vi "movimentacao_cin_inv_bezier_2_com_sensor_att.vi"() -> ()   [LabVIEW 2017]
doc: "The myRIO Project template acquires acceleration data from the onboard accelerometer and displays the changes of acceleration values in a waveform chart."
uses:
  <vilib>/Analysis/Matrix/Datatypes/RealMatrix.ctl
  <vilib>/myRIO/Instrument Drivers/Onboard IO/I2C/typedefs/I2C User Configuration.ctl
  <vilib>/myRIO/Instrument Drivers/Onboard IO/I2C/typedefs/I2C Transfer Rate.ctl
  <vilib>/myRIO/Instrument Drivers/Onboard IO/PWM/typedefs/PWM Reference.ctl
  <vilib>/myRIO/Common/Instrument Driver Framework/Utilities/typedefs/myRIO Generic Hardware Reference.ctl
  <vilib>/myRIO/Common/Instrument Driver Framework/Utilities/typedefs/Hardware Version Enum.ctl
  <vilib>/myRIO/Common/Instrument Driver Framework/Utilities/typedefs/myRIO v1.0 Reference.ctl
  <vilib>/myRIO/Common/Instrument Driver Framework/Utilities/typedefs/Generic FPGA Reference.ctl
  <vilib>/myRIO/Common/Instrument Driver Framework/myRIO v1.0/PWM/typedefs/PWM Channels Enum.ctl
  <vilib>/myRIO/Instrument Drivers/Onboard IO/PWM/typedefs/PWM Configuration.ctl
  <vilib>/userdefined/High Color/nirio_resource_hc.ctl
  <vilib>/myRIO/Instrument Drivers/Onboard IO/I2C/typedefs/I2C Reference.ctl
  <vilib>/myRIO/Common/Instrument Driver Framework/myRIO v1.0/I2C/typedefs/I2C Channels Enum.ctl
  <vilib>/myRIO/Instrument Drivers/Onboard IO/I2C/typedefs/I2C Configuration.ctl
  <vilib>/myRIO/Common/Instrument Driver Framework/myRIO v1.0/I2C/vis/myRIO v1.1 Open I2C.vi
  <vilib>/myRIO/Common/Instrument Driver Framework/myRIO v1.0/PWM/vis/myRIO v1.1 Open PWM.vi
  <vilib>/myRIO/Common/Instrument Driver Framework/Utilities/vis/Validate Channels.vi
  <vilib>/myRIO/Common/Instrument Driver Framework/myRIO v1.0/I2C/vis/myRIO v1.0 Reserve I2C.vi
  <vilib>/myRIO/Common/Instrument Driver Framework/myRIO v1.0/I2C/vis/myRIO v1.0 Close I2C.vi
  <vilib>/myRIO/Common/Instrument Driver Framework/myRIO v1.0/PWM/vis/myRIO v1.0 Reserve PWM.vi
  <vilib>/myRIO/Instrument Drivers/Onboard IO/PWM/vis/Set Duty Cycle and Frequency.vi
  <vilib>/myRIO/Common/Instrument Driver Framework/myRIO v1.0/PWM/vis/myRIO v1.0 Close PWM.vi
  <vilib>/myRIO/Common/Instrument Driver Framework/myRIO v1.0/I2C/vis/myRIO v1.0 Build MUX Configuration I2C.vi
  <vilib>/myRIO/Common/Instrument Driver Framework/myRIO v1.0/Resource Manager/vis/myRIO v1.0 Reserve Channel List.vi
  <vilib>/myRIO/Common/Instrument Driver Framework/myRIO v1.0/I2C/vis/myRIO v1.0 Unreserve I2C.vi
  <vilib>/myRIO/Common/Instrument Driver Framework/myRIO v1.0/PWM/vis/myRIO v1.0 Build MUX Configuration PWM.vi
  <vilib>/myRIO/Common/Instrument Driver Framework/myRIO v1.0/PWM/vis/myRIO v1.0 Unreserve PWM.vi
  <vilib>/myRIO/Common/Instrument Driver Framework/myRIO v1.0/Resource Manager/vis/myRIO v1.0 Create Configuration List.vi
  <vilib>/myRIO/Common/Instrument Driver Framework/myRIO v1.0/Resource Manager/vis/myRIO v1.0 Reserve Channel.vi
  <vilib>/myRIO/Common/Instrument Driver Framework/myRIO v1.0/Resource Manager/vis/myRIO v1.0 Unreserve Channel.vi
  <vilib>/myRIO/Common/Instrument Driver Framework/myRIO v1.0/Resource Manager/vis/myRIO v1.0 Unreserve Channel List.vi
  <vilib>/myRIO/Common/Instrument Driver Framework/myRIO v1.0/Resource Manager/vis/myRIO v1.0 Build Mutex Name.vi
  <vilib>/Utility/VariantDataType/GetNumericInfo.vi
  <vilib>/Utility/error.llb/Error Cluster From Error Code.vi
  <vilib>/myRIO/Common/Instrument Driver Framework/myRIO v1.0/myRIO v1.1 Open.vi
  <vilib>/myRIO/Common/Instrument Driver Framework/Utilities/vis/IO Manager.vi
  <vilib>/myRIO/Common/Instrument Driver Framework/Utilities/vis/Configuration Manager.vi
  <vilib>/myRIO/Common/Instrument Driver Framework/myRIO v1.0/Resource Manager/vis/myRIO v1.0 Configure IO.vi
  <vilib>/myRIO/Common/Instrument Driver Framework/myRIO v1.0/myRIO v1.0 Close.vi
  <vilib>/myRIO/Common/Instrument Driver Framework/myRIO v1.0/PWM/vis/myRIO v1.0 Write PWM.vi
  <vilib>/myRIO/Common/Instrument Driver Framework/myRIO v1.0/PWM/vis/myRIO v1.0 Shutdown PWM.vi
  <vilib>/myRIO/Common/Instrument Driver Framework/myRIO v1.0/I2C/vis/myRIO v1.0 Configure I2C.vi
  <vilib>/myRIO/Common/Instrument Driver Framework/myRIO v1.0/I2C/vis/myRIO v1.0 Shutdown I2C.vi
  <vilib>/myRIO/Instrument Drivers/Onboard IO/PWM/vis/myRIO PWM Open.xnode
  <vilib>/myRIO/Instrument Drivers/Onboard IO/I2C/vis/myRIO I2C Open.xnode
  <vilib>/myRIO/Instrument Drivers/Onboard IO/PWM/PWM.lvlib
  <vilib>/myRIO/Instrument Drivers/Onboard IO/I2C/I2C.lvlib
  <vilib>/Analysis/Matrix/NI_Matrix.lvlib
panel:
  out "x-y":i32
  out "Fim_manipulacao":bool
  out "indexador 2":i32
  in  "Time Target (s) 2":dbl=0.2 format="%#_13g"
  out "x < y?":bool
  out "reconheceu 2":bool
  out "Local_da_peca 2":i8
  out "Elapsed Time (s) 2":dbl
  out "Time has Elapsed 2":bool
  out "x .and. y?":bool
  out "var aux":bool=TRUE
  in  "OK Button":bool
  out "Detectou 2":bool
  out "mean out":dbl
  in  "y":dbl=135.0
  out "PARAR ESTEIRA":bool
  out "reconheceu":bool
  out "x .and. y? 2":bool
  out "Detectou":bool
  in  "Duty Cycle Abert 2":dbl=0.08 format="%#_13g"
  out "Local_da_peca":i8
  out "PARAR 2":bool
  out "spreadsheet string":string
  out "error out 2":errorcluster
  out "init status 2":bool
  out "did_timeout 2":bool
  out "dt 2":u32
  out "Waveform Chart 2":u16(graph)
  out "Range (cm)":u16
  out "objeto":bool
  out "distancaia 2":dbl format="%0.2f"
  out "result string":string
  out "iterador":u32
  out "number of rows":i32
  out "matrix":T1
  out "subarray":dbl[](array[numeric])
  out "appended array 2":dbl[](array[numeric])
  out "POS_E_ORIEN_HOME":dbl[](array[numeric])
  out "ANG_POSI_E_ORIEN_HOME":dbl[](array[numeric])
  out "CURRENT POSITIONS OF THE MOTORS":dbl[](array[numeric])
  in  "angulo_garra":dbl(knob) scale=-180.0..180.0
  in  "Duty Cycle Abert":dbl=0.04 format="%#_13g"
  out "Actuator 2":bool
  in  "Actuator":bool
  in  "Conveyor speed (mm/s)":dbl(slide)=200.0 step=1.0 scale=0.0..350.0
  out "indexador":i32
  out "Manipulando":bool
  out "Está em Home":bool
  out "Posicao_desejada":bool
  in  "Home":bool
  in  "error in (no error)":errorcluster
  in  "PARAR":bool
  in  "POSITION VECTOR":dbl[](array[numeric])
  # "ROTINA DE CONTROLE DO PROTÓTIPO DE FMS"
  # "COMANDO DE POSI敲O\nATUAL DOS MOTORES"
  # "OPERATION STATUS"
  # "ÂNGULOS DE JUNTAS"
  # "THETA 1"
  # "MOTOR 1"
  # "HOME"
  # "THETA 2"
  # "MOTOR 2"
  # "POSI敲O DESEJADA"
  # "THETA 3"
  # "MOTOR 3"
  # "OBJETO DETECTADO"
  # "THETA 4"
  # "MOTOR 4"
  # "MANIPULANDO"
  # "THETA 5"
  # "MOTOR 5"
  # "ESTEIRA PARADA"
  # "MOTOR 6"
  # "ATUADOR"
  # "VELOCIDADE DA ESTEIRA (mm/s)"
  # "0,042"
  # "SCL- CINZA - 32\nSDA - ROXO - 34\nTERRA - BRANCO\nVCC - PRETO"
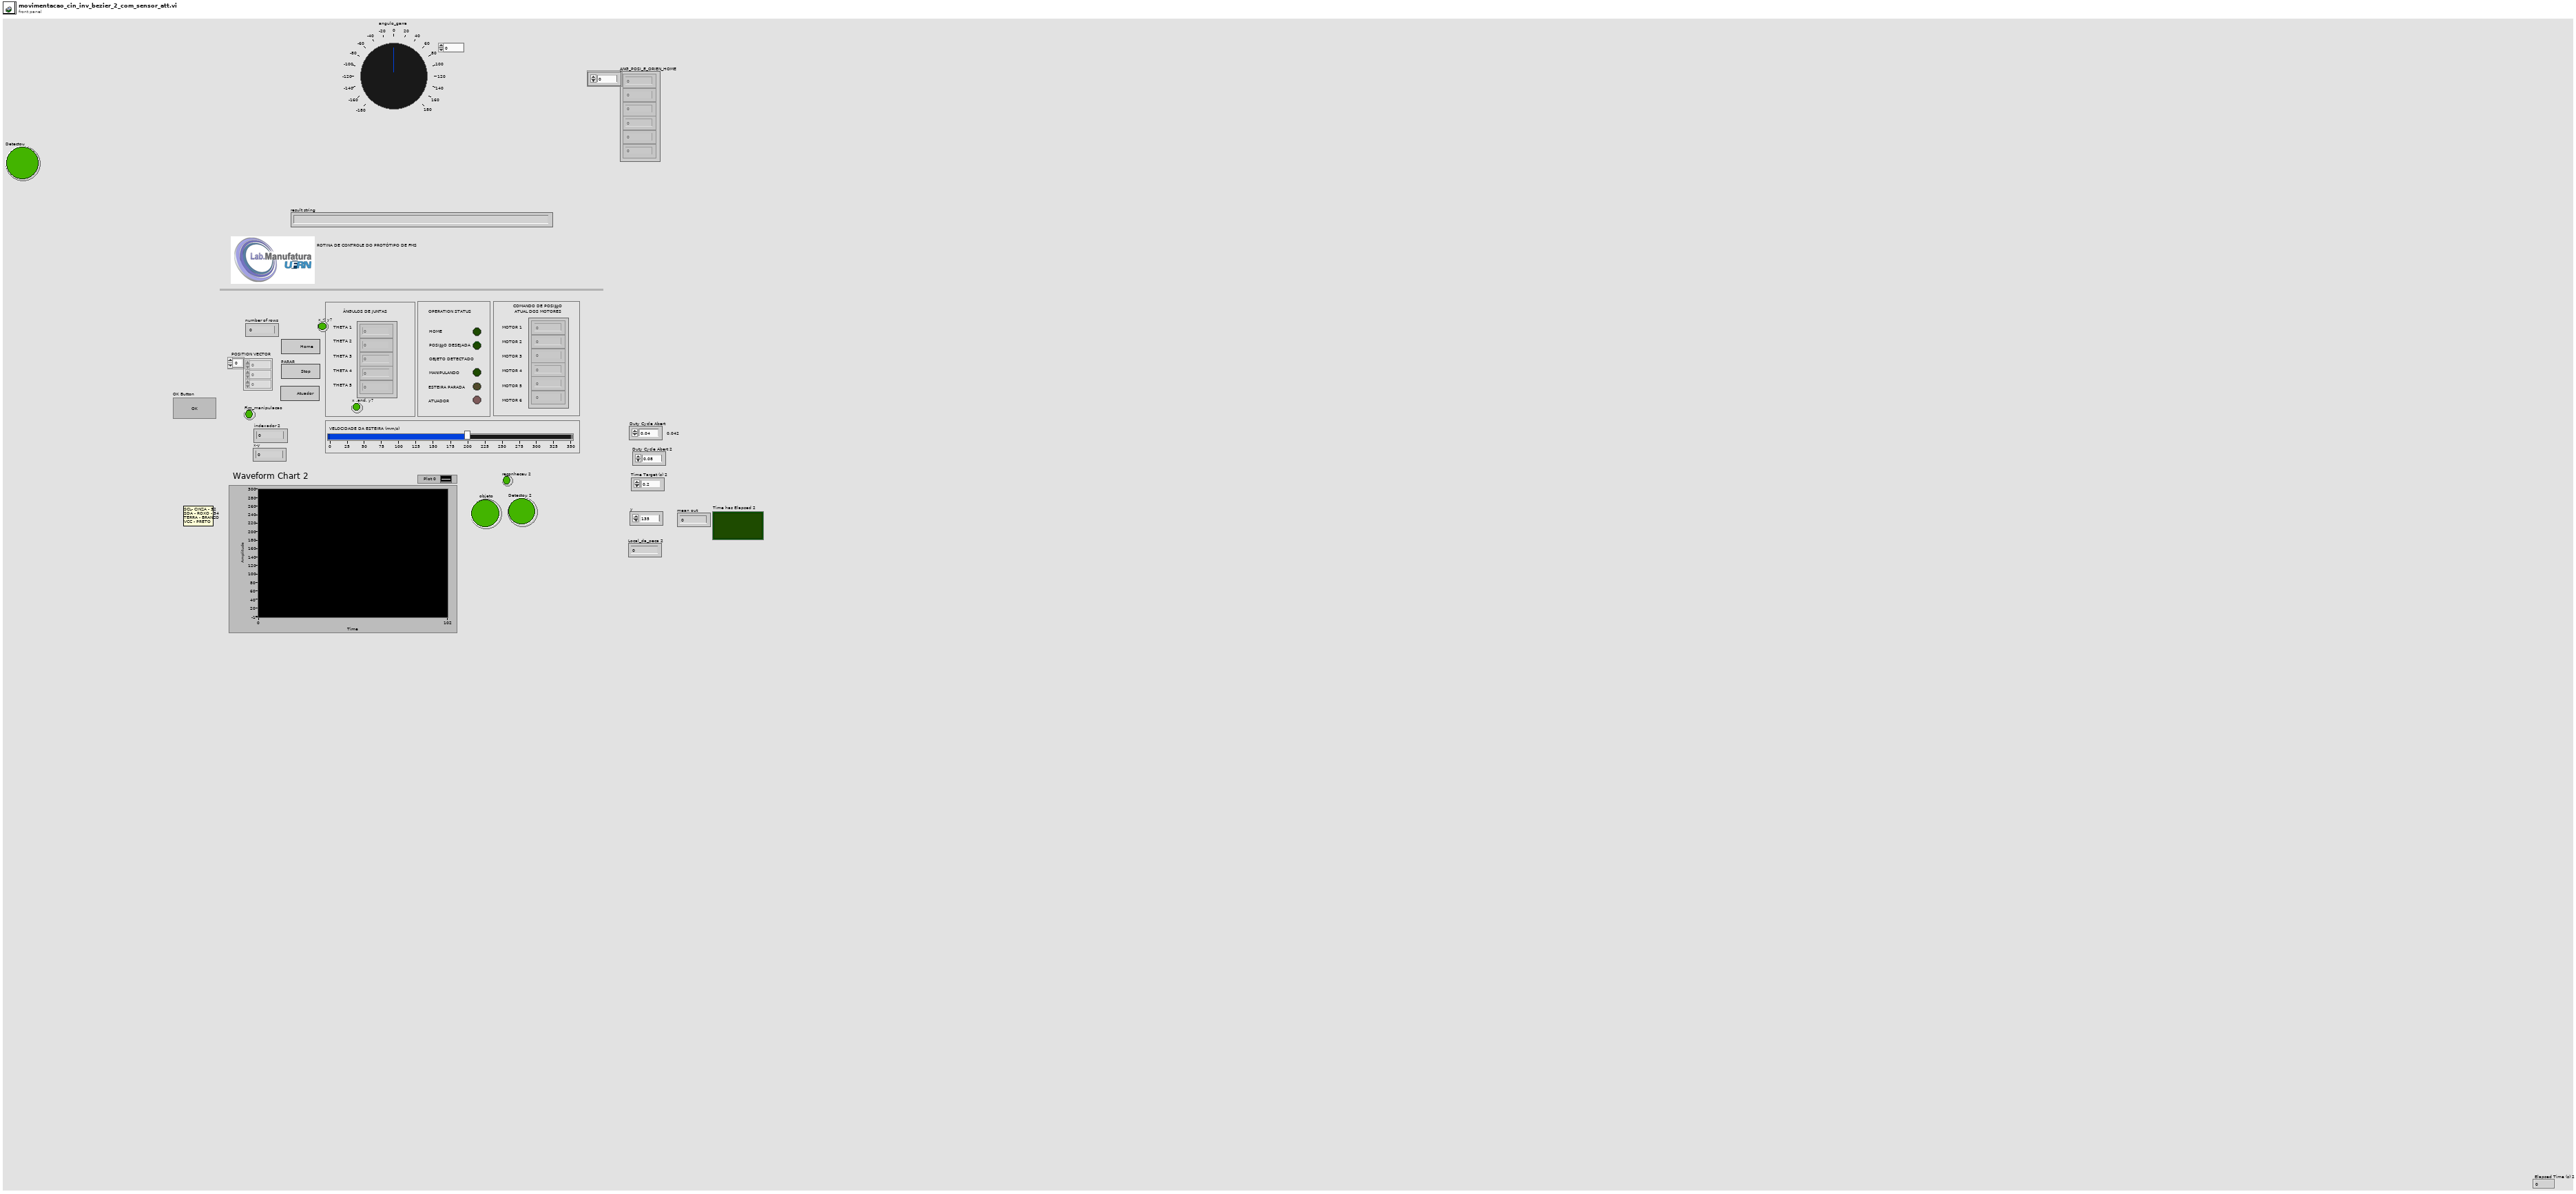
[diagram p1: front panel]
types:
  T1 = typedef "NI_Matrix.lvlib/RealMatrix.ctl" = dbl[][]
  T2 = typedef "I2C.lvlib/I2C User Configuration.ctl" = cluster{"I2C Transfer Rate":T3}
  T3 = typedef "I2C.lvlib/I2C Transfer Rate.ctl" = enum16{"Standard mode (100 kbps)", "Fast mode (400 kbps)"}
  T4 = cluster{"theta 1":dbl, "theta 2":dbl, "theta 3":dbl, "theta5":dbl, "theta4":dbl}
  T5 = typedef "nirio_resource_hc.ctl" = tag
  T6 = typedef "Hardware Version Enum.ctl" = enum16{"Unknown", "myRIO-1900", "myRIO-1950", "roboRIO", "NI ELVIS RIO CM"}
  T7 = typedef "PWM.lvlib/PWM Reference.ctl" = cluster{"myRIO Reference":T8, "PWM Channels Enum":T11, "PWM Configuration":T12}
  T8 = typedef "myRIO Generic Hardware Reference.ctl" = cluster{"myRIO Model":T6, "myRIO Hardware Reference":T9}
  T9 = typedef "myRIO v1.0 Reference.ctl" = cluster{"Generic FPGA Reference":T10, "Allow multiple opens":bool}
  T10 = typedef "Generic FPGA Reference.ctl" = refnum<k20>
  T11 = typedef "PWM Channels Enum.ctl" = enum16{"Not Connected", "C/PWM0", "C/PWM1", "A/PWM0", "A/PWM1", "A/PWM2", "B/PWM0", "B/PWM1", "B/PWM2", "PWM/PWM0", "PWM/PWM1", "PWM/PWM2", "PWM/PWM3", "PWM/PWM4", "PWM/PWM5", "PWM/PWM6", "PWM/PWM7", "PWM/PWM8", "PWM/PWM9"}
  T12 = typedef "PWM.lvlib/PWM Configuration.ctl" = cluster{"Frequency":dbl, "Duty Cycle":dbl}
  T13 = typedef "I2C.lvlib/I2C Reference.ctl" = cluster{"myRIO Reference":T8, "I2C Channels Enum":T14, "I2C Configuration":T15}
  T14 = typedef "I2C Channels Enum.ctl" = enum16{"Not Connected", "A/I2C", "B/I2C", "I2C/I2C"}
  T15 = typedef "I2C.lvlib/I2C Configuration.ctl" = cluster{"I2C Transfer Rate":T3}
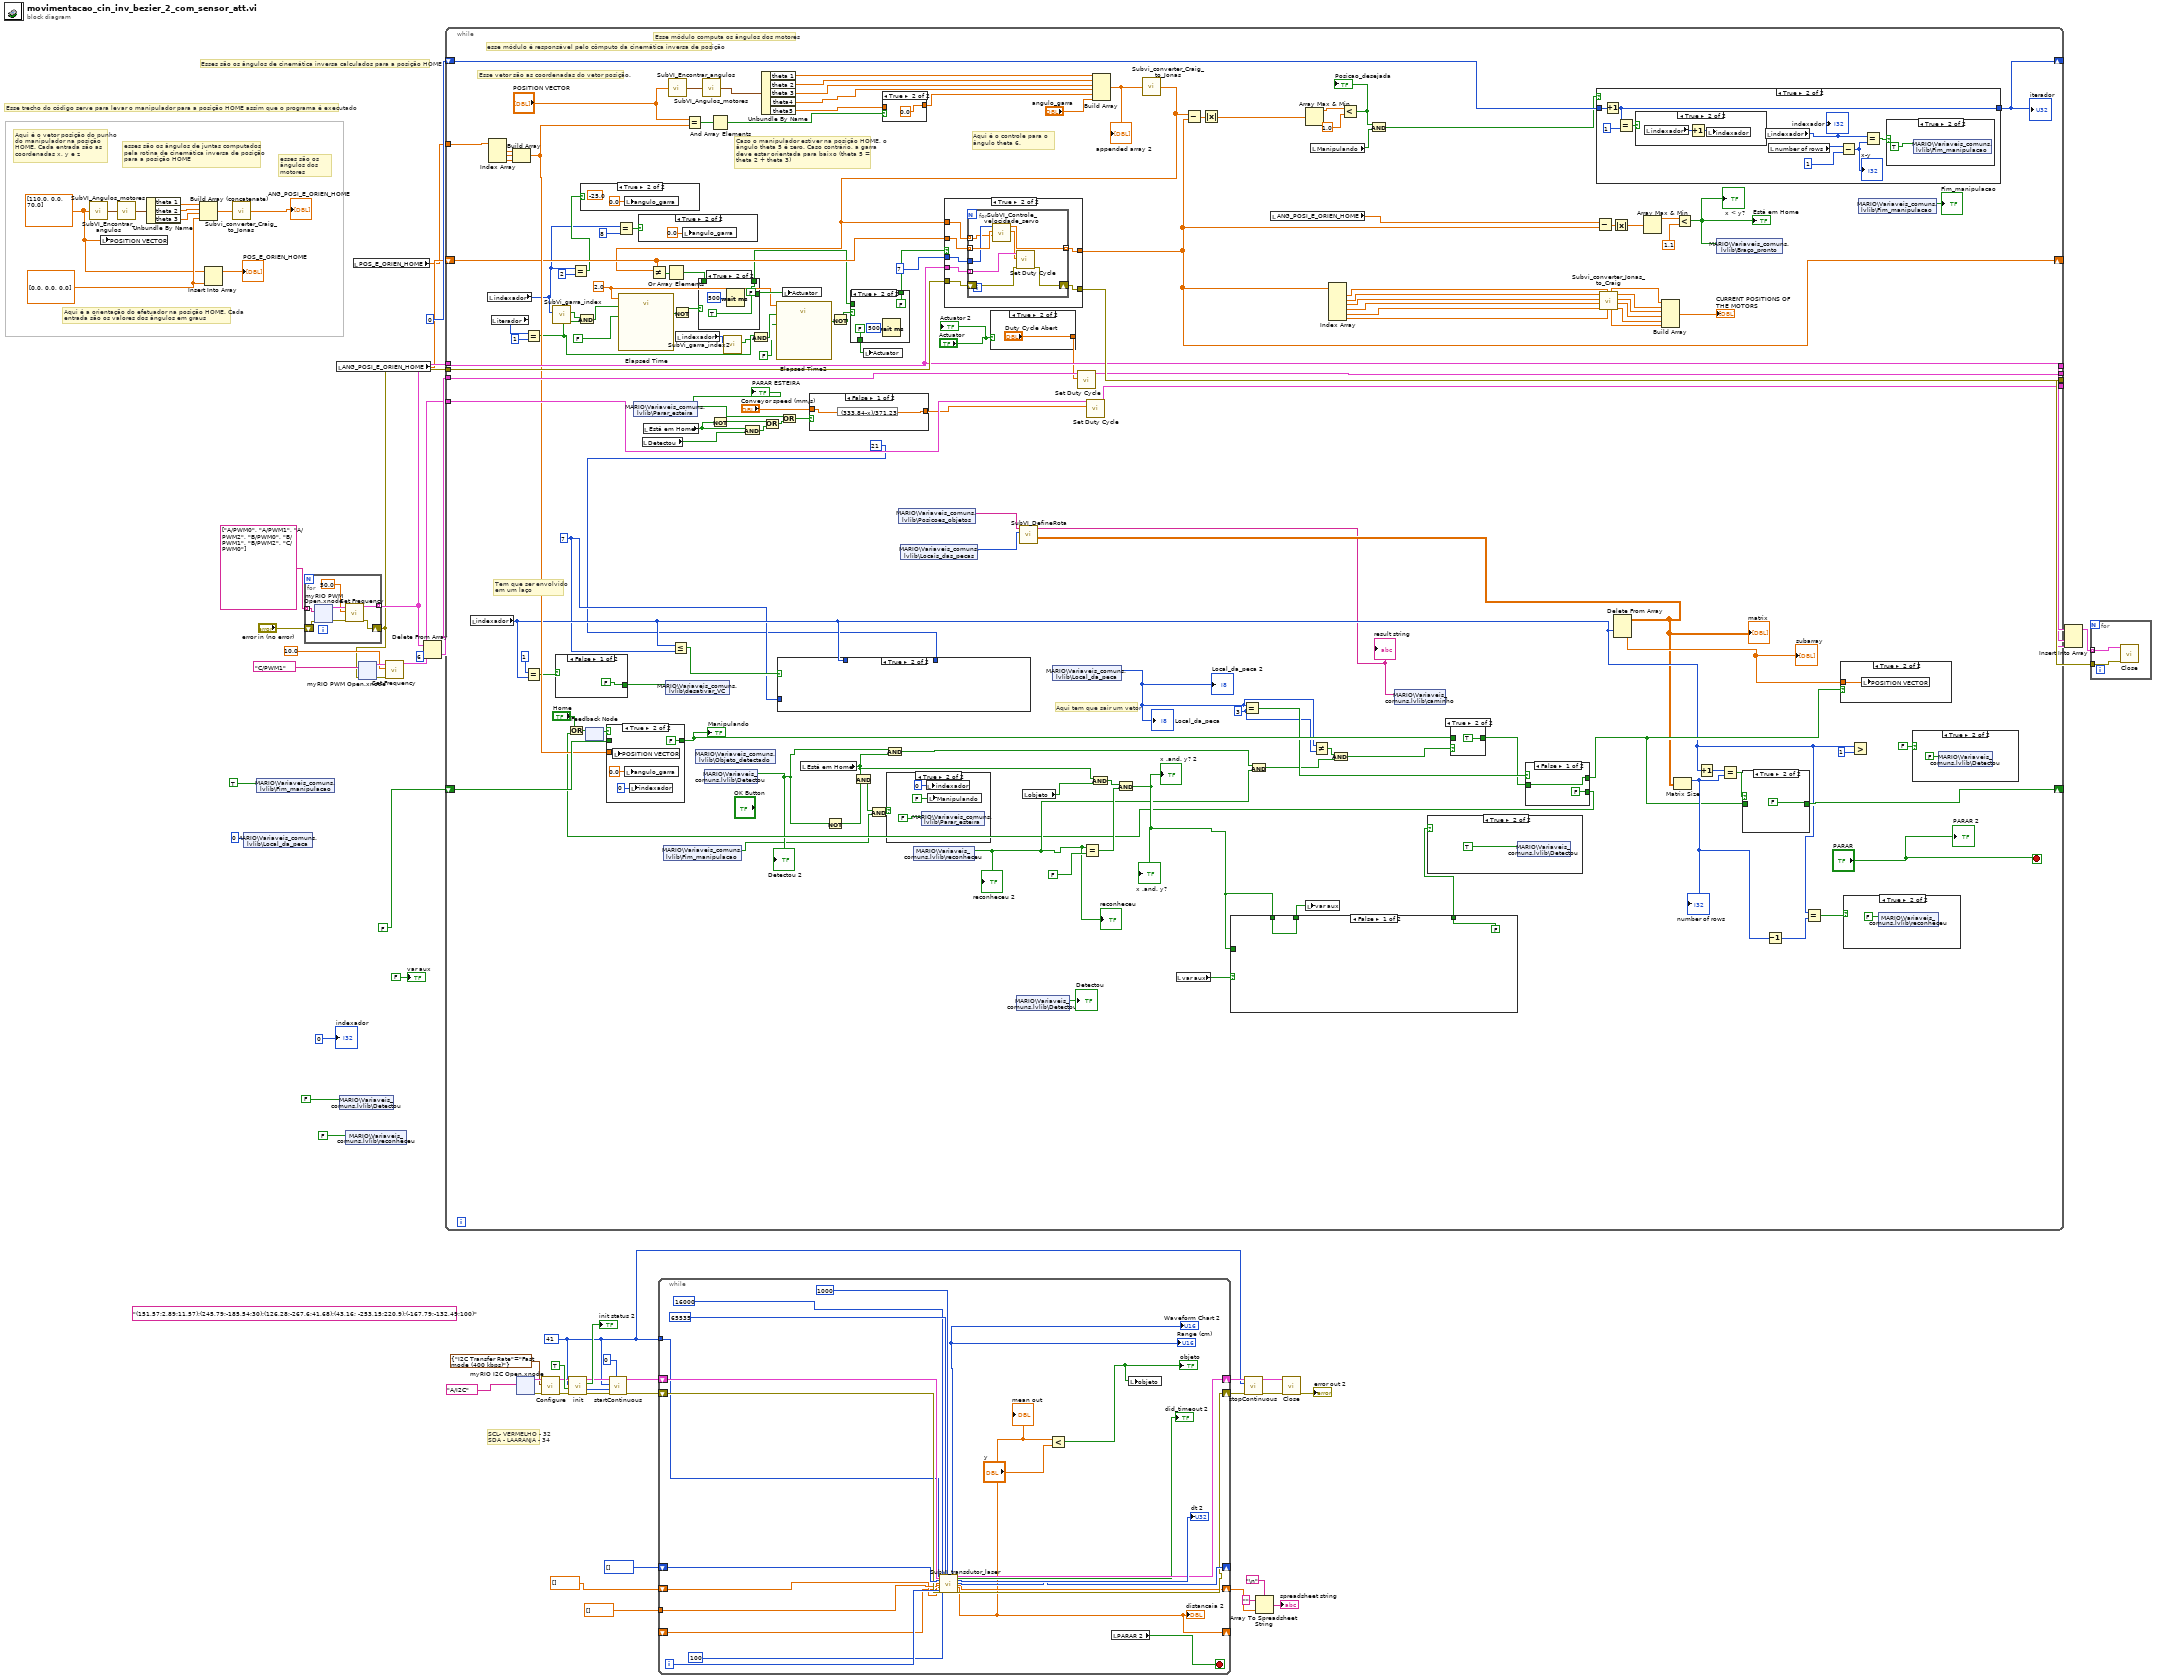
[diagram p0: block diagram]
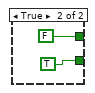
[diagram p2: hidden frame]
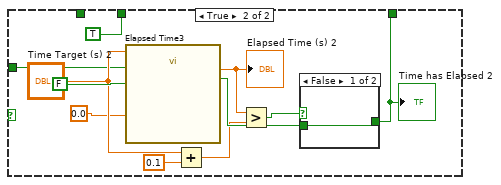
[diagram p3: hidden frame]
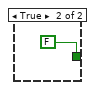
[diagram p4: hidden frame]
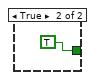
[diagram p8: hidden frame]
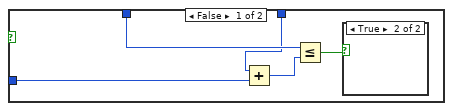
[diagram p11: hidden frame]
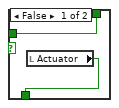
[diagram p13: hidden frame]
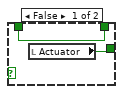
[diagram p14: hidden frame]
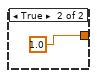
[diagram p16: hidden frame]
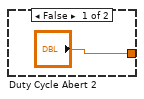
[diagram p17: hidden frame]
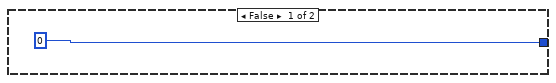
[diagram p20: hidden frame]
diagram:
  w13 = u8 41
  (unwired) "(151,57;2,89;11,57);(245,79;-185,54;30);(126,28;-267,6;41,68);(43,16; -253,15;220,9);(-167,79;-132,49;100)" ("String 2")
  w40 = dbl[] [0.0, 0.0, 0.0] ("vetor_P")
  w3 = dbl[] [110.0, 0.0, 70.0] ("vetor_P")
  # "esses são os ângulos dos motores"
  # "esses são os ângulos de juntas computados pela rotina de cinemática inversa de posição para a posição HOME"
  # "Esses são os ângulos de cinemática inversa calculados para a posição HOME"
  # "Aqui é a orientação do efetuador na posição HOME. Cada entrada são os valores dos ângulos em graus"
  # "Aqui é o vetor posição do punho do manipulador na posição HOME. Cada entrada são as coordenadas x, y e z"
  # "Esse trecho do código serve para levar o manipulador para a posição HOME assim que o programa é executado"
  # "SCL- VERMELHO - 32\nSDA - LAARANJA - 34"
  n1 = call "SubVI_Encontrar_angulos.vi"("vetor_P"=w3) -> ("ângulos de Juntas"=w35:T4)
  n2 = local write "POSITION VECTOR"(w3) -> ()
  n3 = call "SubVI_Angulos_motores.vi"("input cluster"=w35) -> ("output cluster"=w34:T4)
  n4 = Unbundle By Name(w34) -> ("theta 1"=w44:dbl, "theta 2"=w43:dbl, "theta 3"=w42:dbl)
  n5 = Build Array (concatenate)(w44, w43, w42, w40) -> (w37:dbl[])
  n6 = Insert Into Array(array=w3, new element=w40) -> (→"POS_E_ORIEN_HOME":dbl[])  [unwired: 1 in]
  n7 = call "Subvi_converter_Craig_to_Jonas.vi"("array"=w37) -> ("appended array"=→"ANG_POSI_E_ORIEN_HOME":dbl[])
  n8 = shared-variable "MARIO\\Variaveis_comuns.lvlib\\Local_da_peca"(i8 0 ("Local_da_peca")) -> ()  [unwired: 1 in, 1 out]
  n9 = shared-variable "MARIO\\Variaveis_comuns.lvlib\\Fim_manipulacao"(TRUE) -> ()  [unwired: 1 in, 1 out]
  n10 = for {
    tunnel: tag[] ["A/PWM0", "A/PWM1", "A/PWM2", "B/PWM0", "B/PWM1", "B/PWM2", "C/PWM0"] -> [w67] mode=indexing
    tunnel: [w66] -> w57 mode=indexing
    shift-right: [w65] -> w46
    shift-left: "error in (no error)" -> [w64]
    n11 = xnode ("myRIO PWM Open.xnode")("error in (no error)"=w64, "Channel Name"=w67) -> ("error out"=w68:errorcluster, "PWM Ref Out"=w70:T7)  [unwired: 1 in]
    n12 = call <vilib>:"Set Frequency.vi"("error in (no error)"=w68, "Frequency [Hz]"=50.0, "PWM Ref In"=w70) -> ("error out"=w65:errorcluster, "PWM Ref Out"=w66:T7)  [unwired: 6 in]
  }
  n13 = local read "ANG_POSI_E_ORIEN_HOME"() -> (w41:dbl[])
  n14 = shared-variable "MARIO\\Variaveis_comuns.lvlib\\Detectou"(FALSE ("Detectou")) -> ()  [unwired: 1 in, 1 out]
  n15 = shared-variable "MARIO\\Variaveis_comuns.lvlib\\reconheceu"(FALSE ("reconheceu")) -> ()  [unwired: 1 in, 1 out]
  n16 = local read "POS_E_ORIEN_HOME"() -> (w38:dbl[])
  n17 = xnode "myRIO PWM Open.xnode"("error in (no error)"=w46, "Channel Name"=tag "C/PWM1") -> ("error out"=w50:errorcluster, "PWM Ref Out"=w51:T7)  [unwired: 1 in]
  n18 = call <vilib>:"Set Frequency.vi"("error in (no error)"=w50, "Frequency [Hz]"=10.0, "PWM Ref In"=w51) -> ("PWM Ref Out"=w47:T7)  [unwired: 6 in, 1 out]
  n19 = Delete From Array(array=w57, index=6) -> (deleted portion=w55:T7)  [unwired: 1 in, 1 out]
  n20 = while {
    tunnel: [w232] -> w63
    shift-right: [w172] -> _
    shift-left: w41 -> [w164]
    tunnel: w46 -> [w230]
    tunnel: w57 -> [w229]
    tunnel: [w229] -> w54
    shift-right: [w162] -> _
    shift-left: FALSE -> [w216]
    shift-right: [w224] -> _
    shift-left: u32 0 ("ms to wait (braço)") -> [w223]
    tunnel: w55 -> [w211]
    tunnel: [w210] -> w53
    tunnel: w47 -> [w208]
    tunnel: [w204] -> w45
    tunnel: w38 -> [w177]
    stop <- "PARAR" stop-if-true
    w100 = i64 7 ("número de pontos que a matriz deve retornar (nº de divisões + 1)")
    w113 = i8 3 ("y")
    w150 = 2.0 ("Time Target (s)")
    # "Tem que ser envolvido \nem um laço"
    # "Aqui tem que sair um vetor"
    # "Aqui é o controle para o ângulo theta 6."
    # "Caso o manipulador estiver na posição HOME, o ângulo theta 5 é zero. Caso contrário, a garra deve estar orientada para baixo (theta 5 = theta 2 + theta 3)"
    # "Esse módulo computa os ângulos dos motores"
    # "esse módulo é responsável pelo cômputo da cinemática inversa de posição"
    # "Esse vetor são as coordenadas do vetor posição."
    n21 = local read "indexador"() -> (w101:i32)
    n22 = local read "indexador"() -> (w89:i32)
    n23 = Index Array(array=w177) -> (element #1=w180:dbl, element #2=w179:dbl, element #3=w178:dbl)  [unwired: 3 in]
    n24 = local read "iterador"() -> (w160:u32)
    n25 = Build Array(w180, w179, w178) -> (w176:dbl[])
    n26 = Equal?(x=w160, y=u32 1) -> (x = y?=w152:bool)
    n27 = Equal?(x=1, y=w101) -> (x = y?=w137:bool)
    n28 = call "SubVi_garra_index.vi"("Indexador"=w89) -> ("garra_index"=w90:bool)  [unwired: 10 in]
    n29 = case shown="False" w137 {
      tunnel: [FALSE TRUE] -> w136
      frame False {
      }
      frame True {
      }
    }
    n30 = Equal?(x=w89, y=2) -> (x = y?=w141:bool)
    n31 = And(x=w90, y=w152) -> (x .and. y?=w158:bool)
    n32 = case shown="True" w141 {
      frame False {
      }
      frame True {
        (unwired) -25.0 ("angulo_garra")
        n33 = local write "angulo_garra"(0.0 ("angulo_garra")) -> ()
      }
    }
    n34 = feedback #1() -> (w104:bool)  [unwired: 1 in]
    n35 = case shown="True" w104 {
      tunnel: w176 -> [_ w307]
      tunnel: w216 -> [w303 _]
      tunnel: [w303 FALSE ("Manipulando")] -> w171
      frame False {
      }
      frame True {
        n36 = local write "POSITION VECTOR"(w307) -> ()
        n37 = local write "angulo_garra"(0.0 ("angulo_garra")) -> ()
        n38 = local write "indexador"(0 ("indexador")) -> ()
      }
    }
    "Manipulando" <- w171
    n39 = Equal?(x=w89, y=8) -> (x = y?=w139:bool)
    n40 = call "Elapsed Time"("Time Target (s)"=w150, "Reset"=w158, "Auto Reset"=FALSE) -> ("Time has Elapsed"=w156:bool)  [unwired: 9 in, 7 out]
    n41 = shared-variable "MARIO\\Variaveis_comuns.lvlib\\Parar_esteira"() -> (w125:bool)  [unwired: 1 in, 1 out]
    "PARAR ESTEIRA" <- w125
    n42 = case shown="True" w139 {
      frame False {
      }
      frame True {
        n43 = local write "angulo_garra"(0.0 ("angulo_garra")) -> ()
      }
    }
    n44 = local read "Detectou"() -> (w124:bool)
    n45 = local read "Está em Home"() -> (w200:bool)
    n46 = shared-variable "MARIO\\Variaveis_comuns.lvlib\\Fim_manipulacao"() -> (w92:bool)  [unwired: 1 in, 1 out]
    n47 = shared-variable "MARIO\\Variaveis_comuns.lvlib\\desativar_VC"(w136) -> ()  [unwired: 1 in, 1 out]
    n48 = call "SubVI_Encontrar_angulos.vi"("vetor_P"="POSITION VECTOR") -> ("ângulos de Juntas"=w169:T4)
    n49 = Less Or Equal?(x=w101, y=w100) -> (x <= y?=w143:bool)
    n50 = Not(x=w156) -> (.not. x?=w155:bool)
    n51 = local read "indexador"() -> (w87:i32)
    n52 = Equal?(x="POSITION VECTOR", y=w176) -> (x = y?=w214:bool[])
    n53 = shared-variable "MARIO\\Variaveis_comuns.lvlib\\Objeto_detectado"() -> ()  [unwired: 1 in, 2 out]
    n54 = call "SubVI_Angulos_motores.vi"("input cluster"=w169) -> ("output cluster"=w168:T4)
    n55 = shared-variable "MARIO\\Variaveis_comuns.lvlib\\Detectou"() -> (w102:bool)  [unwired: 1 in, 1 out]
    "Detectou 2" <- w102
    n56 = Not(x=w200) -> (.not. x?=w201:bool)
    n57 = And Array Elements(Boolean array=w214) -> (logical AND=w213:bool)
    n58 = call "SubVi_garra_index2.vi"("Indexador"=w87) -> ("garra_index"=w88:bool)  [unwired: 10 in]
    n59 = And(x=w200, y=w124) -> (x .and. y?=w202:bool)
    n60 = And(x=w152, y=w88) -> (x .and. y?=w151:bool)
    n61 = Unbundle By Name(w168) -> ("theta 1"=w185:dbl, "theta 2"=w184:dbl, "theta 3"=w183:dbl, "theta4"=w167:dbl, "theta5"=w166:dbl)
    n62 = Or(x=w201, y=w202) -> (x .or. y?=w199:bool)
    n63 = call "Elapsed Time2"("Time Target (s)"=w150, "Reset"=w151, "Auto Reset"=FALSE) -> ("Time has Elapsed"=w149:bool)  [unwired: 9 in, 7 out]
    n64 = case shown="True" w143 {
      tunnel: w101 -> [w264 _]
      tunnel: i64 21 ("número de pontos que a matriz deve retornar (nº de divisões + 1)") -> [w262 _]
      tunnel: w100 -> [w261 _]
      frame False {
        n65 = Add(x=w262, y=w261) -> (x+y=w260:i64)
        n66 = Less Or Equal?(x=w264, y=w260) -> (x <= y?=w263:bool)
        n67 = case shown="True" w263 {
          frame False {
          }
          frame True {
          }
        }
      }
      frame True {
      }
    }
    n68 = Or(x=w125, y=w199) -> (x .or. y?=w205:bool)
    n69 = local read "Está em Home"() -> (w135:bool)
    n70 = case shown="False" w205 {
      tunnel: [w277 1.0 ("Duty Cycle")] -> w207
      tunnel: "Conveyor speed (mm/s)" -> [w276 _]
      frame False {
        n71 = expression code="(333.84-x)/371.23"(w276) -> (w277:dbl)
      }
      frame True {
      }
    }
    n72 = Not(x=w102) -> (.not. x?=w174:bool)
    n73 = Not(x=w149) -> (.not. x?=w148:bool)
    n74 = And(x=w135, y=w174) -> (x .and. y?=w93:bool)
    n75 = And(x=w93, y=w92) -> (x .and. y?=w94:bool)
    n76 = case shown="True" w213 {
      tunnel: [w281 0.0 ("theta5")] -> w182
      tunnel: w166 -> [w281 _]
      frame False {
      }
      frame True {
      }
    }
    n77 = And(x=w102, y=w135) -> (x .and. y?=w116:bool)
    n78 = case shown="True" w94 {
      frame False {
      }
      frame True {
        n79 = shared-variable "MARIO\\Variaveis_comuns.lvlib\\Parar_esteira"(FALSE) -> ()  [unwired: 1 in, 1 out]
        n80 = local write "indexador"(0 ("indexador")) -> ()
        n81 = local write "Manipulando"(FALSE ("Manipulando")) -> ()
      }
    }
    n82 = shared-variable "MARIO\\Variaveis_comuns.lvlib\\Posicoes_objetos"() -> (w97:string[])  [unwired: 1 in, 1 out]
    n83 = shared-variable "MARIO\\Variaveis_comuns.lvlib\\Locais_das_pecas"() -> (w98:u16[])  [unwired: 1 in, 1 out]
    n84 = shared-variable "MARIO\\Variaveis_comuns.lvlib\\reconheceu"() -> (w117:bool)  [unwired: 1 in, 1 out]
    "reconheceu" <- w117
    "reconheceu 2" <- w117
    n85 = case shown="True" "Actuator" {
      tunnel: ["Duty Cycle Abert 2" "Duty Cycle Abert"] -> w209
      frame False {
      }
      frame True {
      }
    }
    n86 = shared-variable "MARIO\\Variaveis_comuns.lvlib\\Detectou"() -> (→"Detectou":bool)  [unwired: 1 in, 1 out]
    n87 = call "SubVI_DefineRota.vi"("Destino_obj"=w98, "Pos_obj"=w97) -> ("Matriz de pontos"=w96:T1, "Caminho"=w95:string)  [unwired: 8 in]
    "matrix" <- w96
    "result string" <- w95
    n88 = local read "objeto"() -> (w134:bool)
    n89 = shared-variable "MARIO\\Variaveis_comuns.lvlib\\Local_da_peca"() -> (w114:i8)  [unwired: 1 in, 1 out]
    "Local_da_peca" <- w114
    "Local_da_peca 2" <- w114
    n90 = call <vilib>:"Set Duty Cycle.vi"("Duty Cycle"=w209, "PWM Ref In"=w211) -> ("PWM Ref Out"=w210:T7)  [unwired: 7 in, 1 out]
    n91 = Equal?(x=w117, y=FALSE) -> (x = y?=w131:bool)
    n92 = call <vilib>:"Set Duty Cycle.vi"("Duty Cycle"=w207, "PWM Ref In"=w208) -> ("PWM Ref Out"=w204:T7)  [unwired: 7 in, 1 out]
    n93 = And(x=w135, y=w134) -> (x .and. y?=w133:bool)
    n94 = Build Array(w185, w184, w183, w167, w182, "angulo_garra") -> (w123:dbl[])
    "appended array 2" <- w123
    n95 = And(x=w133, y=w131) -> (x .and. y?=w121:bool)
    "x .and. y? 2" <- w121
    "x .and. y?" <- w121
    n96 = call "Subvi_converter_Craig_to_Jonas.vi"("array"=w123) -> ("appended array"=w122:dbl[])
    n97 = Not Equal?(x=w122, y=w164) -> (x != y?=w228:bool[])
    n98 = Or Array Elements(Boolean array=w228) -> (logical OR=w154:bool)
    n99 = case shown="True" w155 {
      tunnel: [w271 FALSE] -> w146
      tunnel: w154 -> [w271 _]
      tunnel: [w270 TRUE ("Actuator")] -> w153
      frame False {
        n100 = local read "Actuator"() -> (w270:bool)
      }
      frame True {
        n101 = Wait (ms)(milliseconds to wait=u32 500) -> ()  [unwired: 1 out]
      }
    }
    n102 = local write "Actuator"(w153) -> ()
    n103 = case shown="True" w148 {
      tunnel: [w266 FALSE ("Actuator")] -> w147
      tunnel: w146 -> [w265 _]
      tunnel: [w265 FALSE] -> w145
      frame False {
        n104 = local read "Actuator"() -> (w266:bool)
      }
      frame True {
        n105 = Wait (ms)(milliseconds to wait=u32 500) -> ()  [unwired: 1 out]
      }
    }
    n106 = local write "Actuator"(w147) -> ()
    n107 = case shown="True" w145 {
      tunnel: [w308 w316] -> w232
      tunnel: w230 -> [w308 w315]
      tunnel: w229 -> [_ w314]
      tunnel: w164 -> [w309 w313]
      tunnel: [w309 w311] -> w172
      tunnel: u32 7 ("ms to wait (braço)") -> [_ w312]
      tunnel: w122 -> [_ w310]
      frame False {
      }
      frame True {
        n108 = for {
          tunnel: w314 -> [w322] mode=indexing
          tunnel: w313 -> [w321] mode=indexing
          tunnel: w312 -> [w319]
          tunnel: [w318] -> w311 mode=indexing
          tunnel: w310 -> [w317] mode=indexing
          shift-right: [w324] -> w316
          shift-left: w315 -> [w323]
          n109 = call "SubVI_Controle_velocidade_servo.vi"("Posição Desejada"=w317, "Posição"=w321, "milliseconds to wait"=w319) -> ("Duty Cycle"=w320:dbl, "Posição"=w318:dbl)  [unwired: 7 in]
          n110 = call <vilib>:"Set Duty Cycle.vi"("error in (no error)"=w323, "Duty Cycle"=w320, "PWM Ref In"=w322) -> ("error out"=w324:errorcluster)  [unwired: 6 in, 1 out]
        }
      }
    }
    n111 = local read "var aux"() -> (w119:bool)
    n112 = Subtract(x=w122, y=w172) -> (x-y=w227:dbl[])
    n113 = Absolute Value(x=w227) -> (abs(x)=w226:dbl[])
    n114 = case shown="False" w119 {
      tunnel: w121 -> [_ w243]
      tunnel: [w239 TRUE ("var aux")] -> w120
      tunnel: w121 -> [w239 _]
      tunnel: [FALSE ("Time has Elapsed") w240] -> w118
      frame False {
      }
      frame True {
        n115 = call "Elapsed Time3"("Time Target (s)"="Time Target (s) 2", "Reset"=w243, "Auto Reset"=FALSE, "Set Start Time (s)"=0.0) -> ("Elapsed Time (s)"=w242:dbl, "Time has Elapsed"=w248:bool)  [unwired: 8 in, 6 out]
        "Elapsed Time (s) 2" <- w242
        n116 = Add(x="Time Target (s) 2", y=0.1) -> (x+y=w245:dbl)
        n117 = Greater?(x=w242, y=w245) -> (0:w249:bool)
        n118 = case shown="False" w249 {
          tunnel: [w251 FALSE ("Time has Elapsed")] -> w240
          tunnel: w248 -> [w251 _]
          frame False {
          }
          frame True {
          }
        }
        "Time has Elapsed 2" <- w240
      }
    }
    n119 = Equal?(x=w114, y=w113) -> (x = y?=w115:bool)
    n120 = And(x=w116, y=w117) -> (x .and. y?=w111:bool)
    n121 = local read "ANG_POSI_E_ORIEN_HOME"() -> (w181:dbl[])
    n122 = Array Max & Min(array=w226) -> (max value=w175:dbl)  [unwired: 3 out]
    n123 = local write "var aux"(w120) -> ()
    n124 = local read "Manipulando"() -> (w222:bool)
    n125 = Not Equal?(x=w114, y=w113) -> (x != y?=w112:bool)
    n126 = Index Array(array=w172) -> (element #1=w198:dbl, element #2=w197:dbl, element #3=w196:dbl, element #4=w195:dbl, element #5=w194:dbl, element #6=w193:dbl)  [unwired: 6 in]
    n127 = And(x=w112, y=w111) -> (x .and. y?=w110:bool)
    n128 = Less?(x=w175, y=1.0) -> (x < y?=w173:bool)
    "Posicao_desejada" <- w173
    n129 = And(x=w173, y=w222) -> (x .and. y?=w221:bool)
    n130 = shared-variable "MARIO\\Variaveis_comuns.lvlib\\caminho"(w95) -> ()  [unwired: 1 in, 1 out]
    n131 = case shown="True" w118 {
      frame False {
      }
      frame True {
        n132 = shared-variable "MARIO\\Variaveis_comuns.lvlib\\Detectou"(TRUE ("Detectou")) -> ()  [unwired: 1 in, 1 out]
      }
    }
    n133 = case shown="True" w110 {
      tunnel: [w301 TRUE] -> w109
      tunnel: w171 -> [w301 _]
      frame False {
      }
      frame True {
      }
    }
    n134 = case shown="False" w115 {
      tunnel: [w235 FALSE ("y")] -> w108
      tunnel: w109 -> [w235 _]
      tunnel: [FALSE ("y") TRUE ("y")] -> w106
      frame False {
      }
      frame True {
      }
    }
    n135 = Or(x="Home", y=w106) -> (x .or. y?=w105:bool)
    n136 = feedback-in #1(w105) -> ()
    n137 = Subtract(x=w181, y=w172) -> (x-y=w220:dbl[])
    n138 = case shown="True" w221 {
      tunnel: w223 -> [_ w294]
      tunnel: [u32 0 ("ms to wait (braço)") w293] -> w224
      frame False {
      }
      frame True {
        n139 = Increment(x=w294) -> (x+1=w293:u32)
        n140 = Equal?(x=w293, y=u32 1) -> (x = y?=w291:bool)
        n141 = case shown="True" w291 {
          frame False {
          }
          frame True {
            n142 = local read "indexador"() -> (w297:i32)
            n143 = Increment(x=w297) -> (x+1=w296:i32)
            n144 = local write "indexador"(w296) -> ()
          }
        }
        n145 = local read "indexador"() -> (w287:i32)
        "indexador 2" <- w287
        n146 = local read "number of rows"() -> (w289:i32)
        n147 = Subtract(x=w289, y=1) -> (x-y=w286:i32)
        "x-y" <- w286
        n148 = Equal?(x=w287, y=w286) -> (x = y?=w290:bool)
        n149 = case shown="True" w290 {
          frame False {
          }
          frame True {
            n150 = shared-variable "MARIO\\Variaveis_comuns.lvlib\\Fim_manipulacao"(TRUE) -> ()  [unwired: 1 in, 1 out]
          }
        }
      }
    }
    "iterador" <- w224
    n151 = call "Subvi_converter_Jonas_to_Craig.vi"("theta6Jonas"=w193, "theta1Jonas"=w198, "theta5Jonas"=w194, "theta4Jonas"=w195, "theta3Jonas"=w196, "theta2Jonas"=w197) -> ("theta5Craig"=w188:dbl, "theta4Craig"=w189:dbl, "theta3Craig"=w190:dbl, "theta2Craig"=w191:dbl, "theta6Craig"=w187:dbl, "theta1Craig"=w192:dbl)
    n152 = Absolute Value(x=w220) -> (abs(x)=w219:dbl[])
    n153 = Delete From Array(array=w96, index (row)=w101) -> (deleted portion=w163:dbl[])  [unwired: 2 in, 1 out]
    "subarray" <- w163
    n154 = Array Max & Min(array=w219) -> (max value=w218:dbl)  [unwired: 3 out]
    n155 = Build Array(w192, w191, w190, w189, w188, w187) -> (→"CURRENT POSITIONS OF THE MOTORS":dbl[])
    n156 = Matrix Size(0:w96) -> (1:w129:i32)  [unwired: 1 out]
    "number of rows" <- w129
    n157 = Less?(x=w218, y=1.1) -> (x < y?=w203:bool)
    "Está em Home" <- w203
    "x < y?" <- w203
    n158 = Increment(x=w101) -> (x+1=w161:i32)
    n159 = shared-variable "MARIO\\Variaveis_comuns.lvlib\\Braço_pronto"(w203) -> ()  [unwired: 1 in, 1 out]
    n160 = Equal?(x=w161, y=w129) -> (x = y?=w215:bool)
    n161 = case shown="True" w215 {
      tunnel: [w283 FALSE ("Manipulando")] -> w162
      tunnel: w108 -> [w283 _]
      frame False {
      }
      frame True {
      }
    }
    n162 = Decrement(x=w129) -> (x-1=w128:i32)
    n163 = Equal?(x=w101, y=w128) -> (x = y?=w127:bool)
    n164 = case shown="True" w108 {
      tunnel: w163 -> [_ w275]
      frame False {
      }
      frame True {
        n165 = local write "POSITION VECTOR"(w275) -> ()
      }
    }
    n166 = case shown="True" w127 {
      frame False {
      }
      frame True {
        n167 = shared-variable "MARIO\\Variaveis_comuns.lvlib\\reconheceu"(FALSE ("reconheceu")) -> ()  [unwired: 1 in, 1 out]
      }
    }
    n168 = Greater?(x=w101, y=1) -> ()  [unwired: 1 out]
    n169 = shared-variable "MARIO\\Variaveis_comuns.lvlib\\Fim_manipulacao"() -> (→"Fim_manipulacao":bool)  [unwired: 1 in, 1 out]
    n170 = case shown="True" FALSE {
      frame False {
      }
      frame True {
        n171 = shared-variable "MARIO\\Variaveis_comuns.lvlib\\Detectou"(FALSE ("Detectou")) -> ()  [unwired: 1 in, 1 out]
      }
    }
    "Actuator 2" <- "Actuator"
    "PARAR 2" <- "PARAR"
  }
  n172 = xnode "myRIO I2C Open.xnode"("Channel Name"=tag "A/I2C") -> ("error out"=w32:errorcluster, "I2C Ref Out"=w33:T13)  [unwired: 2 in]
  n173 = call <vilib>:"Configure.vi"("error in (no error)"=w32, "I2C User Configuration"=T2 {"I2C Transfer Rate"=enum."Fast mode (400 kbps)"}, "I2C Ref In"=w33) -> ("error out"=w23:errorcluster, "I2C Ref Out"=w24:T13)  [unwired: 7 in]
  n174 = call "init.vi"("error in"=w23, "io_2V8"=TRUE, "Slave Address(7 bit)"=w13, "I2C Ref In"=w24) -> ("error out"=w20:errorcluster, "stop_variable"=w19:u8, "Boolean"=→"init status 2":bool, "I2C Ref Out"=w21:T13)  [unwired: 4 in]
  n175 = call "startContinuous.vi"("period_ms"=u32 0, "error in"=w20, "stop_variable"=w19, "Slave Address(7 bit)"=w13, "I2C Ref In"=w21) -> ("error out"=w27:errorcluster, "I2C Ref Out"=w26:T13)  [unwired: 5 in]
  n176 = while {
    shift-right: [w339] -> w17
    shift-left: w26 -> [w341]
    shift-right: [w338] -> w16
    shift-left: w27 -> [w340]
    tunnel: w13 -> [w336]
    shift-right: [w343] -> _
    shift-left: u16[] [] -> [w344]
    tunnel: dbl[] [] ("array") -> [w332]
    shift-right: [w330] -> w8
    shift-left: dbl[] [] ("array") -> [w331]
    shift-right: [w327] -> _
    shift-left: _ -> [w329]
    i -> [w342]
    stop <- w328 stop-if-true
    n177 = call "SubVI_transdutor_laser.vi"("Numeric Control 2"=w336, "I2C Ref Out in"=w341, "Array in"=w344, "array in"=w331, "array 3"=w332, "mean in"=w329, "Numeric Control 3"=w342, "error in (no error)"=w340, "io_timeout"=u16 16000, "Numeric Control"=100, "y 2"=u16 65535 ("y"), "y"=u16 1000) -> ("Range"=→"Waveform Chart 2" →"Range (cm)":u16, "I2C Ref Out out"=w339:T13, "did_timeout"=→"did_timeout 2":bool, "Numeric Control 4"=→"dt 2":u32, "Array out"=w343:u16[], "array out"=w330:dbl[], "mean out"=w327:dbl, "error out"=w338:errorcluster)  [unwired: 7 in, 1 out]
    "distancaia 2" <- w327
    "mean out" <- w327
    n178 = Less?(x=w327, y="y") -> (x < y?=w325:bool)
    "objeto" <- w325
    n179 = local read "PARAR 2"() -> (w328:bool)
    n180 = local write "objeto"(w325) -> ()
  }
  n181 = call "stopContinuous.vi"("error in"=w16, "Slave Address(7 bit)"=w13, "I2C Ref In"=w17) -> ("error out"=w15:errorcluster, "I2C Ref Out"=w14:T13)  [unwired: 7 in]
  n182 = Array To Spreadsheet String(delimiter (Tab)="\n", array=w8, 3:"" ("format string")) -> (spreadsheet string=→"spreadsheet string":string)
  n183 = call <vilib>:"Close.vi"("error in (no error)"=w15, "I2C Ref In"=w14) -> ("error out"=→"error out 2":errorcluster)  [unwired: 9 in]
  n184 = Insert Into Array(array=w54, new element #1=w53, new element #2=w45) -> (w52:T7[])  [unwired: 1 in]
  n185 = for {
    tunnel: w63 -> [w349]
    tunnel: w52 -> [w348] mode=indexing
    n186 = call <vilib>:"Close.vi"("error in (no error)"=w349, "PWM Ref In"=w348) -> ()  [unwired: 9 in, 1 out]
  }
  "indexador" <- 0
  "var aux" <- FALSE ("var aux")
